vi "Init Observed Values.vi"(11 "Vessel in":refnum<class "Vessel.lvclass">) -> (0 "tau":dbl[](array[numeric]), 1 "y_l":dbl[](array[numeric]), 2 "y":dbl[](array[numeric]), 3 "Vessel out":refnum<class "Vessel.lvclass">)   [LabVIEW 2014, in "Observer Library.lvlib" / "Kalman Filter.lvclass"]
uses:
  Kalman Filter.lvclass
  ROV/Vessel.lvclass
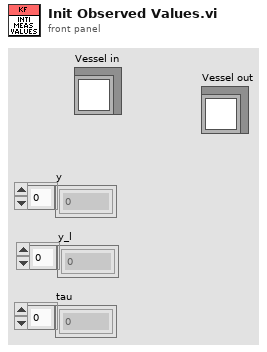
[diagram p1: front panel]
types:
  T1 = cluster{"Measured":cluster{"Eta":dbl[], "Nu":dbl[], "Eta Dot":dbl[], "Nu Dot":dbl[]}, "Estimated":cluster{"Eta":dbl[], "Nu":dbl[], "Eta Dot":dbl[], "Nu Dot":dbl[]}, "Desired":cluster{"Eta":dbl[], "Nu":dbl[], "Eta Dot":dbl[], "Nu Dot":dbl[]}, "Previous Desired":cluster{"Eta":dbl[], "Nu":dbl[], "Eta Dot":dbl[], "Nu Dot":dbl[]}, "tau":dbl[], "Altitude":cluster{"Measured":dbl, "Estimated":dbl, "Desired":dbl, "Previous Desired":dbl, "Approximated":dbl, "grad F":dbl[]}, "rpm":dbl[], "Attitude":cluster{"Theta Measured":dbl[], "Theta Estimated":dbl[], "Omega Measured":dbl[], "Omega Estimated":dbl[], "Gyro Bias":dbl[]}}
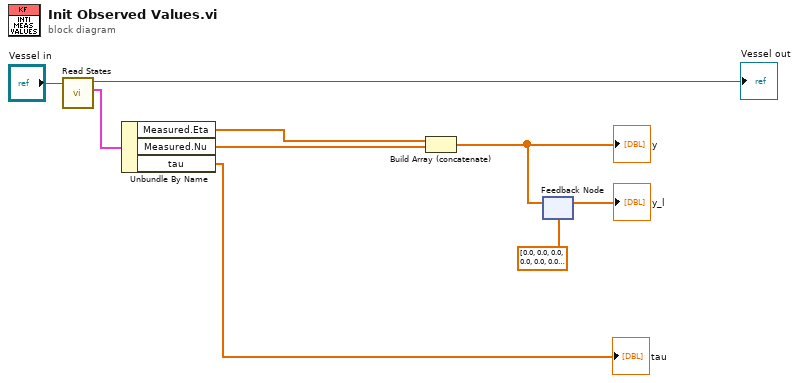
[diagram p0: block diagram]
diagram:
  n1 = call-dynamic "Read States.vi"("Vessel in"="Vessel in") -> ("States"=w4:T1, "Vessel out"=→"Vessel out":refnum<class "Vessel.lvclass">)  [unwired: 8 in, 1 out]
  n2 = Unbundle By Name(w4) -> ("Measured.Eta"=w2:dbl[], "Measured.Nu"=w1:dbl[], "tau"=→"tau":dbl[])
  n3 = Build Array (concatenate)(w2, w1) -> (w7:dbl[])
  "y" <- w7
  n4 = feedback #1(dbl[] [0.0, 0.0, 0.0, 0.0, 0.0, 0.0, 0.0, 0.0, 0.0, 0.0, 0.0, 0.0]) -> (→"y_l":dbl[])
  n5 = feedback-in #1(w7) -> ()
